vi "PH_PPPA_PowerUnit.check Waiting state.vi"(0 "i ref in":refnum<vi>, 5 "error in (no error)":errorcluster) -> (14 "i ref out":refnum<vi>, 17 "Waiting Time (s)":i32, 19 "error out":errorcluster)   [LabVIEW 2014, in "PH_PPPA_PowerUnit.lvlib"]
doc: "This VI calculates the state of the waiting time: if the waiting time is over, \"true\" is indicated. At the waiting time \"0\" appears at \"Waiting Time (s)\" in this case. Otherwise the remaining waiting is indicated in seconds. If an \"9999\" appears, an error occured by checking the waiting time.\n\n\"Required Device(s) off?\" is true if at least one device is even not switched on."
uses:
  PH_PPPA_PowerUnit.lvlib
  CS_Core/BaseSM/BaseSM.lvlib
  CSlibraries-extern/DimLVEvent/LVDimInterface/LVDimInterface.lvlib
  PH_Basics/PH_PowerUnit_BaseClass/PH_PowerUnit_BaseClass.lvlib
  PH_Basics/PH_Common/PH_Common.lvlib
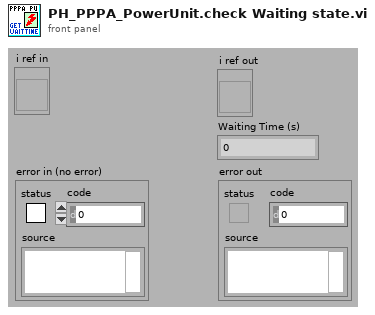
[diagram p1: front panel]
types:
  T1 = typedef "PH_PowerUnit_BaseClass.lvlib/PH_PowerUnit_BaseClass.i attribute.ctl" = cluster{"Constructor finished":bool, "PU":cluster{"In use":bool, "Service ID in use":i32, "GUI Ref":refnum<vi>}, "Enabling":cluster{"State":T2, "GUI Ref":refnum<vi>}, "Timing":cluster{"Last Shot":dbl, "Time between Shots [Sec]":dbl, "Waiting Time over?":bool, "Service ID Waiting Time":i32, "GUI Ref":refnum<vi>, "Instance":cluster{"Status":T3, "linked?":bool, "GUI Ref":refnum<vi>}}, "Sequencer":cluster{"SM State":string, "GUI Ref":refnum<vi>, "linked":bool}, "Subscribed Trendmssgs":cluster{"Tagname":string, "Status":T3, "linked?":bool, "Shot Condition":T3, "GUI Ref":refnum<vi>}[], "PP PU":T4, "Default Voltage (V)":dbl, "GUI Refs":T5, "PSDB data":cluster{"Shot Voltage [V]":dbl, "State TO SM":T6, "Write 2 early":bool}, "State TO SM":T6}
  T2 = typedef "PH_SystemInformation.lvlib/PH_SystemInformationEnabling State.ctl" = i32
  T3 = typedef "PH_StatusHandler.lvlib/PH_StatusHandler.Status.ctl" = i16
  T4 = typedef "PH_PP_Common.lvlib/PH_PP_Common.PUs.ctl" = enum16{"no Info", "PA-19mm-1", "PA-19mm-2", "PA-45mm-PILC", "PA-45mm-MAIN", "MA-PU-1", "MA-PU-2", "MA-PU-3", "MA-PU-4", "MA-PU-5", "MA-PU-6", "MA-FR", "MA-PILC", "PA-45mm-DP"}
  T5 = typedef "PH_PowerUnit_BaseClass.lvlib/PH_PowerUnit_BaseClass.GUI Refs.ctl" = cluster{"Delete Inst":refnum<vi>, "State TO SM":refnum<vi>, "State SM":refnum<vi>, "Fire":refnum<vi>}
  T6 = typedef "PH_PowerUnit_BaseClass.lvlib/PH_PowerUnit_BaseClass.SM States.ctl" = enum16{".", "Stand by", "Switch PU on", "Configure", "Set Default Voltage", "Set STANDBY", "Set READY", "Wait for Shot Cmd", "Open Dump Rods", "Open Ross Relais", "Close Ross Relais", "Switch PSU on", "Switch PSU off", "Charge", "Switch GD Channel on", "Close Dump Rods", "Rods-TO", "RR-TO", "PSU-TO", "Trigger-TO"}
  T7 = typedef "PH_PPPA_PowerUnit.lvlib/PH_PPPA_PowerUnit.i attribute.ctl" = cluster{"GUI Refs":cluster{"Ignitron":refnum<vi>, "Rossrelais":refnum<vi>, "Set Voltage":refnum<vi>, "PSU":refnum<vi>, "EOC":refnum<vi>, "Trigger":refnum<vi>}, "Ignitron":T8, "PSU":T9, "Dump Ross Relais":T10, "Trigger":cluster{"State Device":T3, "linked?":bool}, "Timing Settings":cluster{"Prdc Fast?":bool, "Default Value Periodic Interval":i32, "Mercury on since":dbl, "Warm up Time Mercury [s]":dbl}, "Set Voltage [V]":dbl, "19er Ignitionbox":string}
  T8 = typedef "PH_PP_Common.lvlib/PH_PP_Common.Ignitron Attributes.ctl" = cluster{"State Device":T3, "linked?":bool}
  T9 = typedef "PH_PP_Common.lvlib/PH_PP_Common.PSU Attributes.ctl" = cluster{"lower limit [V]":dbl, "upper limit [V]":dbl, "Voltage set":bool, "State Device":T3, "linked?":bool}
  T10 = typedef "PH_PP_Common.lvlib/PH_PP_Common.Ross Relais Attributes.ctl" = cluster{"State Device":T3, "linked?":bool}
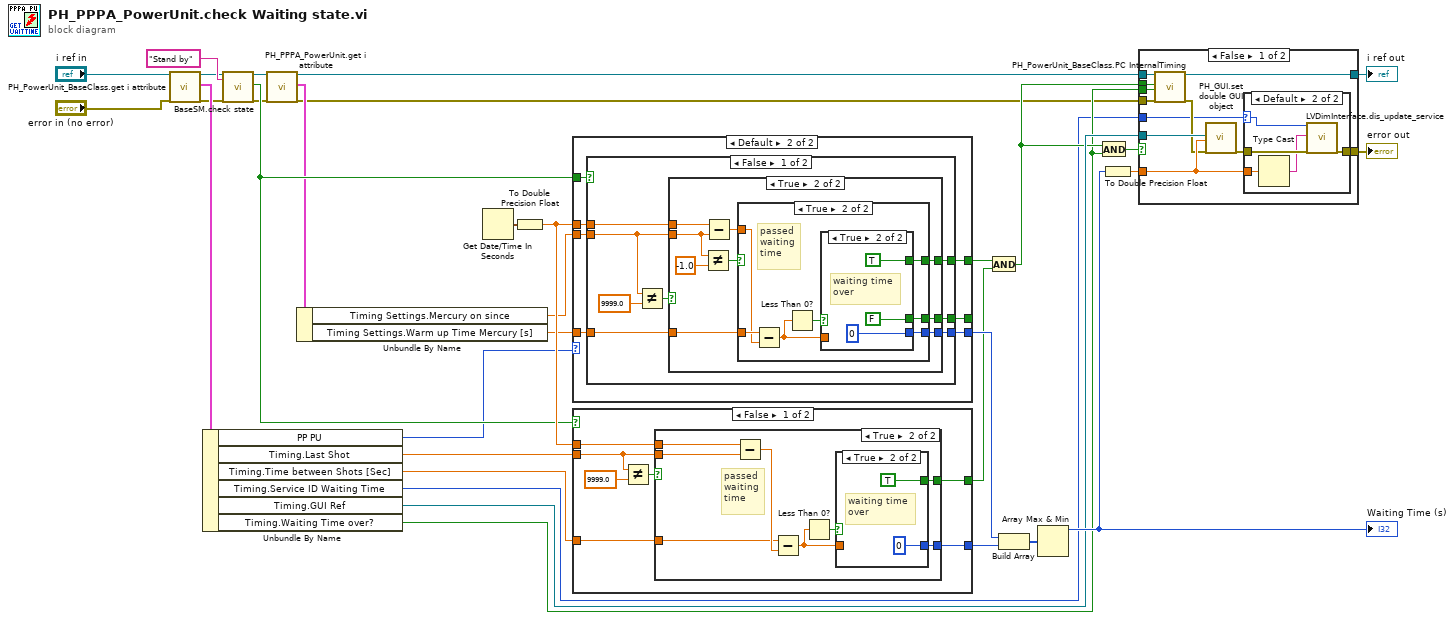
[diagram p0: block diagram]
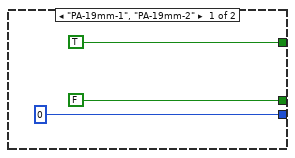
[diagram p4: hidden frame]
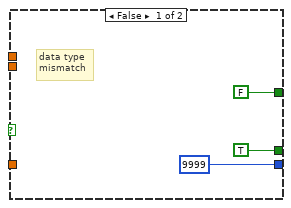
[diagram p5: hidden frame]
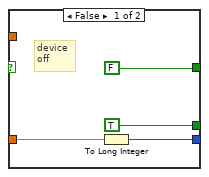
[diagram p6: hidden frame]
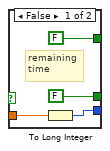
[diagram p7: hidden frame]
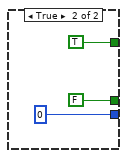
[diagram p8: hidden frame]
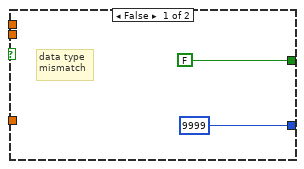
[diagram p9: hidden frame]
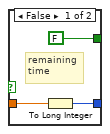
[diagram p10: hidden frame]
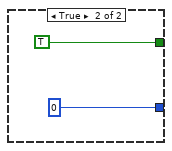
[diagram p11: hidden frame]
diagram:
  n1 = call "PH_PowerUnit_BaseClass.get i attribute.vi"("i ref in"="i ref in", "error in (no error)"="error in (no error)") -> ("i ref out"=w2:refnum<vi>, "i attribute"=w18:T1, "error out"=w1:errorcluster)  [unwired: 15 in]
  n2 = Unbundle By Name(w18) -> ("PP PU"=w4:T4, "Timing.Last Shot"=w5:dbl, "Timing.Time between Shots [Sec]"=w16:dbl, "Timing.Service ID Waiting Time"=w6:i32, "Timing.GUI Ref"=w17:refnum<vi>, "Timing.Waiting Time over?"=w11:bool)
  n3 = call "BaseSM.check state.vi"("i ref in"=w2, "requestedState"="Stand by" ("requested state"), "error in (no error)"=w1) -> ("i ref out"=w15:refnum<vi>, "OK"=w25:bool, "error out"=w22:errorcluster)  [unwired: 11 in, 3 out]
  n4 = call "PH_PPPA_PowerUnit.get i attribute.vi"("i ref in"=w15, "error in (no error)"=w22) -> ("i ref out"=w9:refnum<vi>, "i attribute"=w14:T7, "error out"=w10:errorcluster)  [unwired: 15 in]
  n5 = Unbundle By Name(w14) -> ("Timing Settings.Mercury on since"=w13:dbl, "Timing Settings.Warm up Time Mercury [s]"=w3:dbl)
  n6 = Get Date/Time In Seconds() -> (seconds since 1Jan1904=w31:timestamp)
  n7 = To Double Precision Float(number=w31) -> (double precision float=w30:dbl)
  n8 = case shown="Default" w4 {
    tunnel: w25 -> [_ w43]
    tunnel: [TRUE w42] -> w24
    tunnel: w3 -> [_ w41]
    tunnel: w13 -> [_ w40]
    tunnel: w30 -> [_ w39]
    tunnel: [0 w38] -> w29
    tunnel: [FALSE w37] -> _
    frame "PA-19mm-1", "PA-19mm-2" {
    }
    frame Default {
      n9 = case shown="False" w43 {
        tunnel: [w48 FALSE] -> w37
        tunnel: [w49 TRUE] -> w42
        tunnel: w41 -> [w50 _]
        tunnel: w40 -> [w45 _]
        tunnel: w39 -> [w51 _]
        tunnel: [w47 0] -> w38
        frame False {
          n10 = Not Equal?(x=w45, y=9999.0) -> (x != y?=w46:bool)
          n11 = case shown="True" w46 {
            tunnel: w45 -> [_ w56]
            tunnel: w51 -> [_ w58]
            tunnel: w50 -> [_ w55]
            tunnel: [FALSE w63] -> w49
            tunnel: [TRUE w62] -> w48
            tunnel: [9999 w61] -> w47
            frame False {
              # "data type\nmismatch"
            }
            frame True {
              n12 = Not Equal?(x=w56, y=-1.0) -> (x != y?=w59:bool)
              n13 = Subtract(x=w58, y=w56) -> (x-y=w57:dbl)
              n14 = case shown="True" w59 {
                tunnel: w57 -> [_ w68]
                tunnel: w55 -> [w65 w72]
                tunnel: [FALSE w71] -> w63
                tunnel: [TRUE w70] -> w62
                tunnel: [w64 w69] -> w61
                frame False {
                  # "device \noff"
                  n15 = To Long Integer(number=w65) -> (32bit integer=w64:i32)
                }
                frame True {
                  # "passed\nwaiting\ntime"
                  n16 = Subtract(x=w72, y=w68) -> (x-y=w74:dbl)
                  n17 = Less Than 0?(x=w74) -> (x < 0?=w73:bool)
                  n18 = case shown="True" w73 {
                    tunnel: w74 -> [w78 _]
                    tunnel: [w77 0] -> w69
                    tunnel: [FALSE TRUE] -> w71
                    tunnel: [FALSE FALSE] -> w70
                    frame False {
                      # "remaining\ntime"
                      n19 = To Long Integer(number=w78) -> (32bit integer=w77:i32)
                    }
                    frame True {
                      # "waiting time\nover"
                    }
                  }
                }
              }
            }
          }
        }
        frame True {
        }
      }
    }
  }
  n20 = case "Check Waiting Time" shown="False" w25 {
    tunnel: [w89 TRUE] -> w27
    tunnel: w16 -> [w90 _]
    tunnel: w5 -> [w86 _]
    tunnel: w30 -> [w91 _]
    tunnel: [w88 0] -> w23
    frame False {
      n21 = Not Equal?(x=w86, y=9999.0) -> (x != y?=w87:bool)
      n22 = case shown="True" w87 {
        tunnel: w86 -> [_ w97]
        tunnel: w91 -> [_ w99]
        tunnel: w90 -> [_ w94]
        tunnel: [FALSE w101] -> w89
        tunnel: [9999 w100] -> w88
        frame False {
          # "data type\nmismatch"
        }
        frame True {
          # "passed\nwaiting\ntime"
          n23 = Subtract(x=w99, y=w97) -> (x-y=w98:dbl)
          n24 = Subtract(x=w94, y=w98) -> (x-y=w96:dbl)
          n25 = Less Than 0?(x=w96) -> (x < 0?=w95:bool)
          n26 = case shown="True" w95 {
            tunnel: w96 -> [w104 _]
            tunnel: [w103 0] -> w100
            tunnel: [FALSE TRUE] -> w101
            frame False {
              # "remaining\ntime"
              n27 = To Long Integer(number=w104) -> (32bit integer=w103:i32)
            }
            frame True {
              # "waiting time\nover"
            }
          }
        }
      }
    }
    frame True {
    }
  }
  n28 = And(x=w24, y=w27) -> (x .and. y?=w12:bool)
  n29 = Build Array(w29, w23) -> (w28:i32[])
  n30 = Array Max & Min(array=w28) -> (max value=w19:i32)  [unwired: 3 out]
  "Waiting Time (s)" <- w19
  n31 = And(x=w12, y=w11) -> (x .and. y?=w20:bool)
  n32 = To Double Precision Float(number=w19) -> (double precision float=w21:dbl)
  n33 = case shown="False" w20 {
    tunnel: w10 -> [w112 w126]
    tunnel: [w116 w126] -> w7
    tunnel: w9 -> [w119 w127]
    tunnel: [w118 w127] -> w8
    tunnel: w12 -> [w117 _]
    tunnel: w21 -> [w115 _]
    tunnel: w17 -> [w114 _]
    tunnel: w11 -> [w113 _]
    tunnel: w6 -> [w109 _]
    frame False {
      n34 = call "PH_PowerUnit_BaseClass.PC InternalTiming.vi"("i ref in"=w119, "Waiting Time over? new"=w117, "Waiting Time over? old"=w113, "error in (no error)"=w112) -> ("i ref out"=w118:refnum<vi>, "error out"=w111:errorcluster)  [unwired: 14 in]
      n35 = call "PH_GUI.set double GUI object.vi"("GUI object Ref"=w114, "value"=w115, "error in (no error)"=w111) -> ("error out"=w110:errorcluster)  [unwired: 16 in]
      n36 = case shown="Default" w109 {
        selector: w109 -> [_ w123]
        tunnel: [w120 w124] -> w116
        tunnel: w110 -> [w120 w125]
        tunnel: w115 -> [_ w121]
        frame -1 {
        }
        frame Default {
          n37 = Type Cast(x=w121) -> (*(type *) &x=w122:string)  [unwired: 1 in]
          n38 = call "LVDimInterface.dis_update_service.vi"("my_serviceID"=w123, "data"=w122, "error in (no error)"=w125) -> ("error out"=w124:errorcluster)  [unwired: 14 in, 2 out]
        }
      }
    }
    frame True {
    }
  }
  "i ref out" <- w8
  "error out" <- w7
